vi "JSON time series data to variant.vi"(0 "InfluxDB in":refnum<class "InfluxDB Client.lvclass">, 5 "JSON data":string="[{\"name\":\"testSeries\",\"columns\":[\"time\",\"string\",\"extended\",\"double\",\"single\",\"int64\",\"int32\",\"int16\",\"int8\",\"uint64\",\"uint32\",\"uint16\",\"uint8\",\"boolean\"],\"points\":[[1430144955,\"serverA\",23.4,0,0,0,0,0,0,0,0,0,0,true],[1429280957,\"serverB\",24.5,0,0,0,0,0,0,0,0,0,0,false]]}]", 7 "Schema":variant, 9 "Precision (ms)":T1=enum."milliseconds", 11 "error in (no error)":errorcluster) -> (4 "InfluxDB out":refnum<class "InfluxDB Client.lvclass">, 6 "Data (variant)":variant[](array[variant]), 15 "error out":errorcluster)   [LabVIEW 2015, in "InfluxDB Client.lvclass"]
doc: "Convert time series JSON data defined by a scheme to variant data."
uses:
  InfluxDB Client.lvclass
  Time precision.ctl
  <vilib>/Utility/VariantDataType/Type.ctl
  <userlib>/_OpenG.lib/dictionary/dictionary.llb/Dictionary Update (by scalar value)__ogtk.vi
  <vilib>/LVH/i3 JSON/JSON Parsing/Get Array Value at Index Files/Get Array Value at Index - Object.vi
  <vilib>/LVH/i3 JSON/JSON Parsing/Get Object Parameter Files/Get Object Parameter - String.vi
  <vilib>/LVH/i3 JSON/JSON Parsing/Get Object Parameter Files/Get Object Parameter - Array.vi
  <vilib>/LVH/i3 JSON/JSON Parsing/Get Array Value at Index Files/Get Array Value at Index - String.vi
  <vilib>/LVH/i3 JSON/JSON Parsing/Get Array Value at Index Files/Get Array Value at Index - Array.vi
  <vilib>/LVH/i3 JSON/i3-json.lvlib
  <vilib>/Utility/VariantDataType/VariantType.lvlib
panel:
  out "Columns":string[](array[string])
  out "Name":string
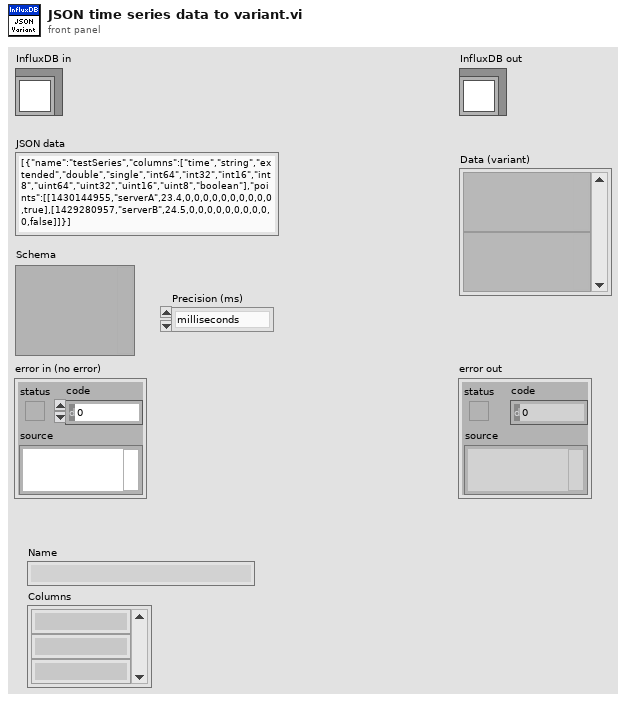
[diagram p1: front panel]
types:
  T1 = typedef "InfluxDB Client.lvclass/Time precision.ctl" = enum16{"seconds", "milliseconds", "microseconds"}
  T2 = typedef "VariantType.lvlib/Type.ctl" = enum8{"Invalid Type", "Void", "I8", "I16", "I32", "I64", "U8", "U16", "U32", "U64", "Single Float", "Double Float", "Extended Float", "Single Complex", "Double Complex", "Extended Complex", "Enum U8", "Enum U16", "Enum U32", "Enum U64", "Single Float With Unit", "Double Float With Unit", "Extended Float With Unit", "Single Complex with Unit", "Double Complex with Unit", "Extended Complex with Unit", "Boolean", "String", "Path", "Picture", "Tag", "Array", "Cluster", "Variant", "LV Variant", "Waveform", "Timestamp", "Digital Waveform", "Digital Data", "ExpressData", "Refnum", "External Data", "VI", "Poly VI", "LabVIEW Class Instance", "Fixed Point"}
  T3 = typedef "Dictionary Object RefNum__ogtk.ctl" = refnum<k1>
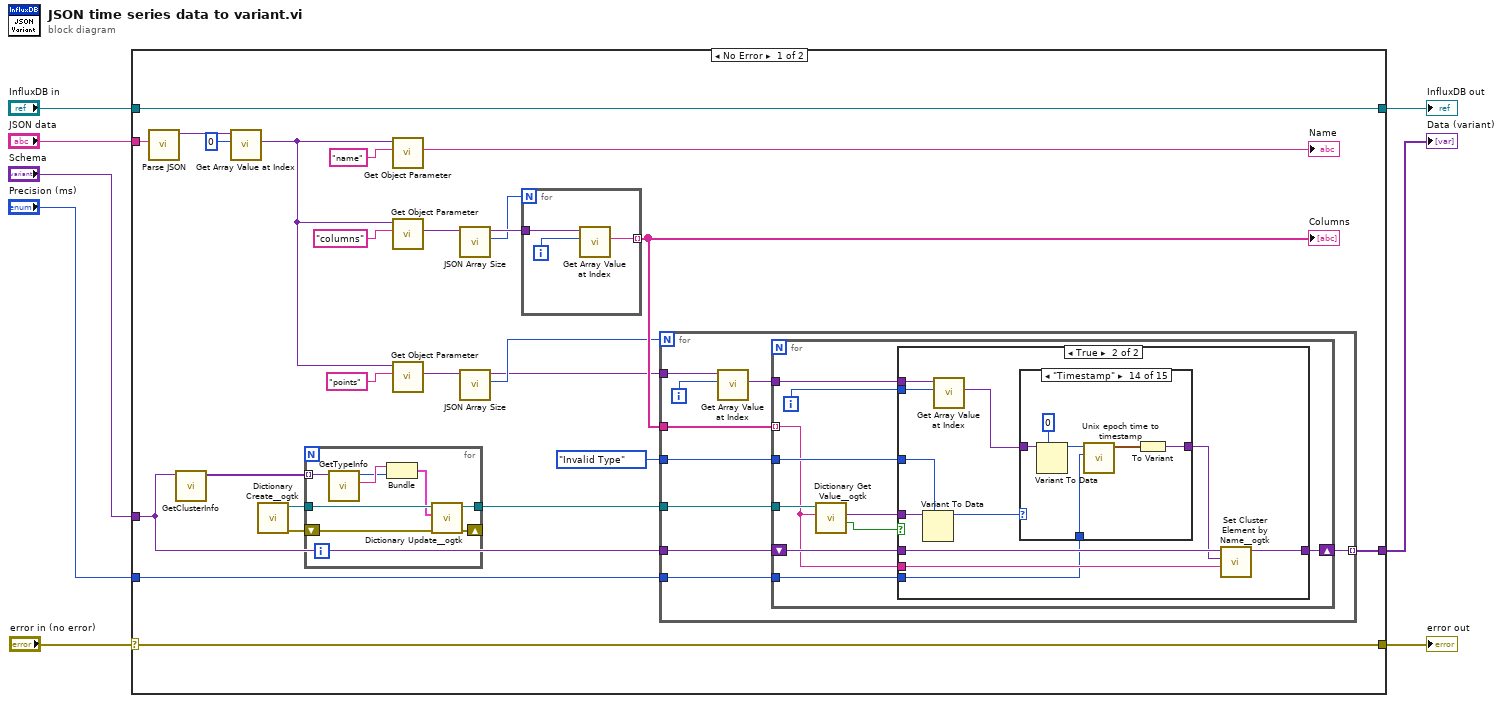
[diagram p0: block diagram]
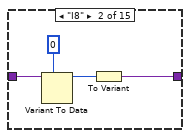
[diagram p4: hidden frame]
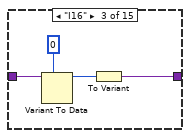
[diagram p5: hidden frame]
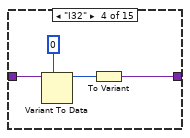
[diagram p6: hidden frame]
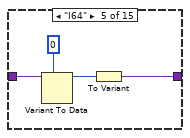
[diagram p7: hidden frame]
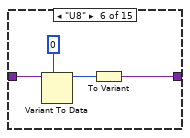
[diagram p8: hidden frame]
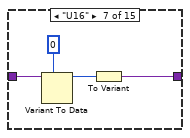
[diagram p9: hidden frame]
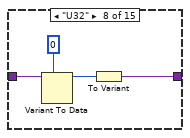
[diagram p10: hidden frame]
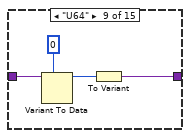
[diagram p11: hidden frame]
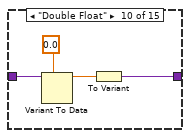
[diagram p12: hidden frame]
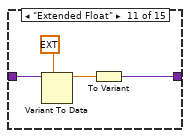
[diagram p13: hidden frame]
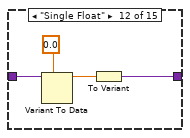
[diagram p14: hidden frame]
diagram:
  n1 = case shown="No Error" "error in (no error)" {
    selector: "error in (no error)" -> [w32 w129]
    tunnel: [w32 w129] -> w7
    tunnel: [w33 w128] -> w5
    tunnel: "InfluxDB in" -> [w33 w128]
    tunnel: "JSON data" -> [w13 _]
    tunnel: "Schema" -> [w12 _]
    tunnel: [w11 _] -> w2
    tunnel: "Precision (ms)" -> [w9 _]
    frame No Error {
      n2 = call <vilib>:"Parse JSON.vi"("JSON String"=w13) -> ("JSON Tree"=w10:variant)  [unwired: 7 in, 3 out]
      n3 = call <vilib>:"GetClusterInfo.vi"("Variant"=w12) -> ("Cluster Elements"=w20:variant[])  [unwired: 9 in, 1 out]
      n4 = call-poly <vilib>:"Get Array Value at Index.vi"("Index"=0, "JSON Tree In (JSON Array)"=w10) -> ("JSON Object"=w19:variant)  [unwired: 6 in, 3 out]
      n5 = call <userlib>:"Dictionary Create__ogtk.vi"() -> ("error out"=w28:errorcluster, "dictionary out"=w27:T3)  [unwired: 10 in]
      n6 = for {
        tunnel: w20 -> [w44] mode=indexing
        tunnel: w27 -> [w43]
        tunnel: [w42] -> w29
        shift-right: [w41] -> _
        shift-left: w28 -> [w40]
        n7 = call <vilib>:"GetTypeInfo.vi"("Variant"=w44) -> ("Name"=w39:string, "Type Enum"=w38:T2)  [unwired: 6 in, 3 out]
        n8 = Bundle("Name"=w39, "Type Enum"=w38) -> (w37:cluster{"Name":string, "Type Enum":T2})  [unwired: 1 in]
        n9 = call-poly <userlib>:"Dictionary Update__ogtk.vi"("error in (no error)"=w40, "key-value"=w37, "dictionary"=w43) -> ("error out"=w41:errorcluster, "dictionary out"=w42:T3)  [unwired: 6 in, 1 out]
      }
      n10 = call-poly <vilib>:"Get Object Parameter.vi"("Parameter Name"="name", "JSON Tree In (JSON Object)"=w19) -> ("String Value"=→"Name":string)  [unwired: 6 in, 3 out]
      n11 = call-poly <vilib>:"Get Object Parameter.vi"("Parameter Name"="columns", "JSON Tree In (JSON Object)"=w19) -> ("JSON Array"=w26:variant)  [unwired: 6 in, 3 out]
      n12 = call-poly <vilib>:"Get Object Parameter.vi"("Parameter Name"="points", "JSON Tree In (JSON Object)"=w19) -> ("JSON Array"=w15:variant)  [unwired: 6 in, 3 out]
      n13 = call <vilib>:"JSON Array Size.vi"("JSON Tree In (JSON Array)"=w26) -> ("Array Size"=w24:i32, "JSON Tree Passthrough (JSON Array)"=w25:variant)  [unwired: 8 in, 1 out]
      n14 = call <vilib>:"JSON Array Size.vi"("JSON Tree In (JSON Array)"=w15) -> ("Array Size"=w17:i32, "JSON Tree Passthrough (JSON Array)"=w16:variant)  [unwired: 8 in, 1 out]
      n15 = for {
        N: w24 -> [_]
        tunnel: w25 -> [w36]
        tunnel: [w34] -> w31 mode=indexing
        i -> [w35]
        n16 = call-poly <vilib>:"Get Array Value at Index.vi"("Index"=w35, "JSON Tree In (JSON Array)"=w36) -> ("String Value"=w34:string)  [unwired: 6 in, 3 out]
      }
      "Columns" <- w31
      n17 = for {
        N: w17 -> [_]
        tunnel: w16 -> [w53]
        tunnel: w12 -> [w50]
        tunnel: [w49] -> w11 mode=indexing
        tunnel: w29 -> [w48]
        tunnel: Type."Invalid Type" ("Type Enum") -> [w47]
        tunnel: w31 -> [w46]
        tunnel: w9 -> [w45]
        i -> [w52]
        n18 = call-poly <vilib>:"Get Array Value at Index.vi"("Index"=w52, "JSON Tree In (JSON Array)"=w53) -> ("JSON Array"=w51:variant)  [unwired: 6 in, 3 out]
        n19 = for {
          tunnel: w51 -> [w62]
          shift-right: [w60] -> w49
          shift-left: w50 -> [w61]
          tunnel: w48 -> [w59]
          tunnel: w47 -> [w57]
          tunnel: w46 -> [w56] mode=indexing
          tunnel: w45 -> [w54]
          i -> [w63]
          n20 = call <userlib>:"Dictionary Get Value__ogtk.vi"("key"=w56, "dictionary"=w59) -> ("found?"=w55:bool, "value"=w58:variant)  [unwired: 6 in, 2 out]
          n21 = case shown="True" w55 {
            tunnel: w63 -> [_ w75]
            tunnel: w62 -> [_ w74]
            tunnel: w61 -> [w64 w73]
            tunnel: [w64 w71] -> w60
            tunnel: w58 -> [_ w69]
            tunnel: w57 -> [_ w68]
            tunnel: w56 -> [_ w66]
            tunnel: w54 -> [_ w65]
            frame False {
            }
            frame True {
              n22 = Variant To Data(type=w68, Variant=w69) -> (data=w67:T2)  [unwired: 1 in, 1 out]
              n23 = call-poly <vilib>:"Get Array Value at Index.vi"("Index"=w75, "JSON Tree In (JSON Array)"=w74) -> ("JSON Object"=w70:variant)  [unwired: 6 in, 3 out]
              n24 = case shown="\"Timestamp\"" w67 {
                tunnel: w70 -> [_ w76 w82 w86 w90 w94 w98 w102 w106 w110 w114 w118 w120 w125 w127]
                tunnel: [_ w77 w80 w84 w88 w92 w96 w100 w104 w108 w112 w116 w120 w123 w127] -> w72
                tunnel: w65 -> [_ _ _ _ _ _ _ _ _ _ _ _ _ w121 _]
                frame Default {
                }
                frame "I8" {
                  n25 = Variant To Data(type=i8 0, Variant=w76) -> (data=w78:i8)  [unwired: 1 in, 1 out]
                  n26 = To Variant(anything=w78) -> (Variant=w77:variant)
                }
                frame "I16" {
                  n27 = Variant To Data(type=i16 0, Variant=w82) -> (data=w81:i16)  [unwired: 1 in, 1 out]
                  n28 = To Variant(anything=w81) -> (Variant=w80:variant)
                }
                frame "I32" {
                  n29 = Variant To Data(type=0, Variant=w86) -> (data=w85:i32)  [unwired: 1 in, 1 out]
                  n30 = To Variant(anything=w85) -> (Variant=w84:variant)
                }
                frame "I64" {
                  n31 = Variant To Data(type=i64 0, Variant=w90) -> (data=w89:i64)  [unwired: 1 in, 1 out]
                  n32 = To Variant(anything=w89) -> (Variant=w88:variant)
                }
                frame "U8" {
                  n33 = Variant To Data(type=u8 0, Variant=w94) -> (data=w93:u8)  [unwired: 1 in, 1 out]
                  n34 = To Variant(anything=w93) -> (Variant=w92:variant)
                }
                frame "U16" {
                  n35 = Variant To Data(type=u16 0, Variant=w98) -> (data=w97:u16)  [unwired: 1 in, 1 out]
                  n36 = To Variant(anything=w97) -> (Variant=w96:variant)
                }
                frame "U32" {
                  n37 = Variant To Data(type=u32 0, Variant=w102) -> (data=w101:u32)  [unwired: 1 in, 1 out]
                  n38 = To Variant(anything=w101) -> (Variant=w100:variant)
                }
                frame "U64" {
                  n39 = Variant To Data(type=u64 0, Variant=w106) -> (data=w105:u64)  [unwired: 1 in, 1 out]
                  n40 = To Variant(anything=w105) -> (Variant=w104:variant)
                }
                frame "Double Float" {
                  n41 = Variant To Data(type=0.0, Variant=w110) -> (data=w109:dbl)  [unwired: 1 in, 1 out]
                  n42 = To Variant(anything=w109) -> (Variant=w108:variant)
                }
                frame "Extended Float" {
                  n43 = Variant To Data(type=ext 0.0, Variant=w114) -> (data=w113:ext)  [unwired: 1 in, 1 out]
                  n44 = To Variant(anything=w113) -> (Variant=w112:variant)
                }
                frame "Single Float" {
                  n45 = Variant To Data(type=sgl 0.0, Variant=w118) -> (data=w117:sgl)  [unwired: 1 in, 1 out]
                  n46 = To Variant(anything=w117) -> (Variant=w116:variant)
                }
                frame "String" {
                }
                frame "Timestamp" {
                  n47 = Variant To Data(type=u64 0, Variant=w125) -> (data=w124:u64)  [unwired: 1 in, 1 out]
                  n48 = call "Unix epoch time to timestamp.vi"("Precision (ms)"=w121, "Unix epoch time"=w124) -> ("Time Stamp"=w122:timestamp)  [unwired: 9 in]
                  n49 = To Variant(anything=w122) -> (Variant=w123:variant)
                }
                frame "Boolean" {
                }
              }
              n50 = call <userlib>:"Set Cluster Element by Name__ogtk.vi"("Element Name (\"\": New Element Data Name)"=w66, "New Element Value"=w72, "Cluster"=w73) -> ("VCluster out"=w71:variant)  [unwired: 6 in, 2 out]
            }
          }
        }
      }
    }
    frame Error {
    }
  }
  "error out" <- w7
  "InfluxDB out" <- w5
  "Data (variant)" <- w2
